vi "6.vi"(11 "Degrees Celcius":dbl) -> (3 "Degrees Fahrenheit":dbl)   [LabVIEW 2015]
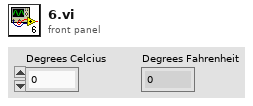
[diagram p1: front panel]
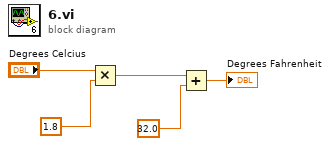
[diagram p0: block diagram]
diagram:
  n1 = Multiply(x="Degrees Celcius", y=1.8) -> (x*y=w3:dbl)
  n2 = Add(x=w3, y=32.0 ("x+y")) -> (x+y=→"Degrees Fahrenheit":dbl)
